vi "Config-Tab Switch.vi"(8 "error in (no error)":errorcluster, 11 "Data Cluster In":T2={"UI Reference"={"All Ctrl's Label's"=[], "ChannelListTree"=refnum, "All Object Ref"=[]}, "Tree Selection"={"Selected Channel"="", "Selected Interface"="", "Selected HW"="", "Tree Root Name"="", "Selected Module"=""}, "Selected File Path"=path "", "Selected HW"={"Slctd Hw Name"=[], "Slctd HW IP"=[]}, "Channel Config Path"=path "", "Interface Data"={"DO Channel's"=[]}, "General Info's"={"Idnentification name"=""}, "Status"="", "Channel Type's"={"Channel Type"=enum."Voltage", "Sub-Type"=enum."Pressure"}, "This VI"=refnum, "Hardware Information "=variant(variant[] [])}) -> (0 "error out":errorcluster, 2 "Config":T1(ring), 3 "Data Cluster Out":T2={"UI Reference"={"All Ctrl's Label's"=[], "ChannelListTree"=refnum, "All Object Ref"=[]}, "Tree Selection"={"Selected Channel"="", "Selected Interface"="", "Selected HW"="", "Tree Root Name"="", "Selected Module"=""}, "Selected File Path"=path "", "Selected HW"={"Slctd Hw Name"=[], "Slctd HW IP"=[]}, "Channel Config Path"=path "", "Interface Data"={"DO Channel's"=[]}, "General Info's"={"Idnentification name"=""}, "Status"="", "Channel Type's"={"Channel Type"=enum."Voltage", "Sub-Type"=enum."Pressure"}, "This VI"=refnum, "Hardware Information "=variant(variant[] [])})   [LabVIEW 2021, in "Configuration.lvlib"]
doc: "<b>Note:</b> This VI was modified by the <b>Validate DQMH Module</b> tool to turn off automatic error handling."
uses:
  Configuration.lvlib
  Module Data--cluster.ctl
  Host-Control's/Configuration UI Reference.ctl
  DO Channel's.ctl
  Config-Channel Type.ctl
  Channel Sub-Type.ctl
  <vilib>/Utility/error.llb/Clear Errors.vi
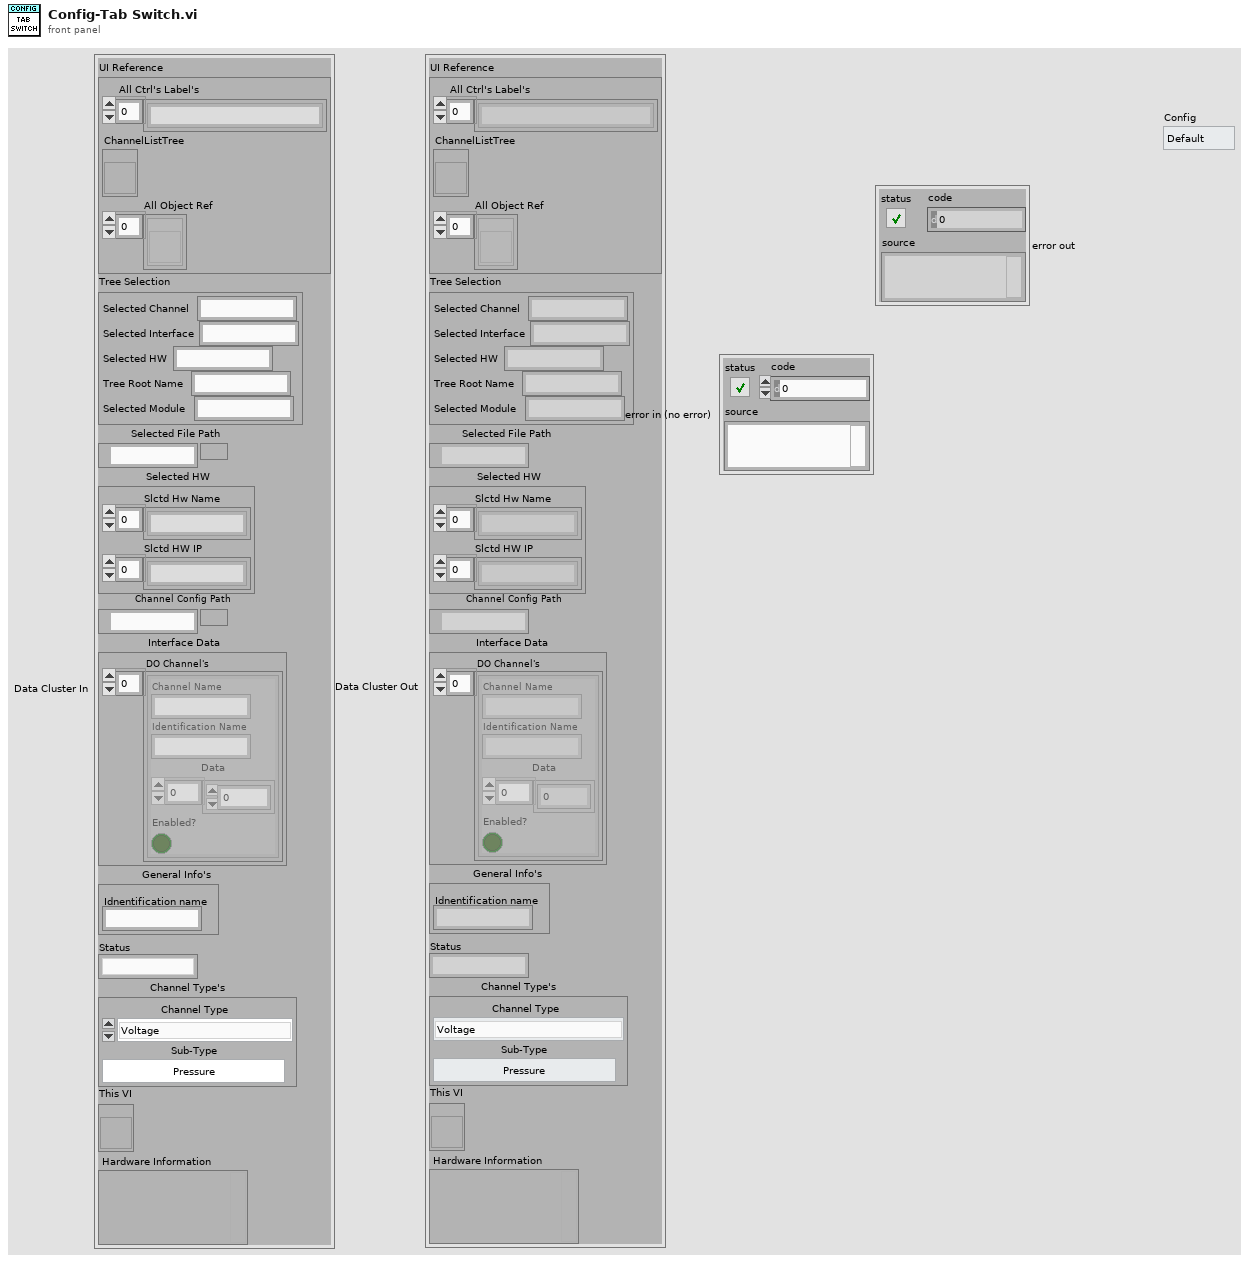
[diagram p1: front panel]
types:
  T1 = enum32{"Default", "Analog Input", "Analog Output", "Digital Input", "Digital Output", "Counter Input", "Counter Output"}
  T2 = typedef "Configuration.lvlib/Module Data--cluster.ctl" = cluster{"UI Reference":T3, "Tree Selection":cluster{"Selected Channel":string, "Selected Interface":string, "Selected HW":string, "Tree Root Name":string, "Selected Module":string}, "Selected File Path":path, "Selected HW":cluster{"Slctd Hw Name":string[], "Slctd HW IP":string[]}, "Channel Config Path":path, "Interface Data":cluster{"DO Channel's":T4}, "General Info's":cluster{"Idnentification name":string}, "Status":string, "Channel Type's":cluster{"Channel Type":T5, "Sub-Type":T6}, "This VI":refnum<vi>, "Hardware Information ":variant}
  T3 = typedef "Configuration UI Reference.ctl" = cluster{"All Ctrl's Label's":string[], "ChannelListTree":refnum<vi>, "All Object Ref":refnum<vi>[]}
  T4 = typedef "Configuration.lvlib/DO Channel's.ctl" = cluster{"Channel Name":string, "Identification Name":string, "Data":u8[], "Enabled?":bool}[]
  T5 = typedef "Configuration.lvlib/Config-Channel Type.ctl" = enum16{"Voltage", "Current", "Thermocouple", "Acclerometer"}
  T6 = typedef "Configuration.lvlib/Channel Sub-Type.ctl" = enum16{"None", "Pressure", "Force"}
  T7 = enum32{"Default", "AI-Voltage", "AI-Current", "AI-ThermoCouple", "AI-Acclerometer"}
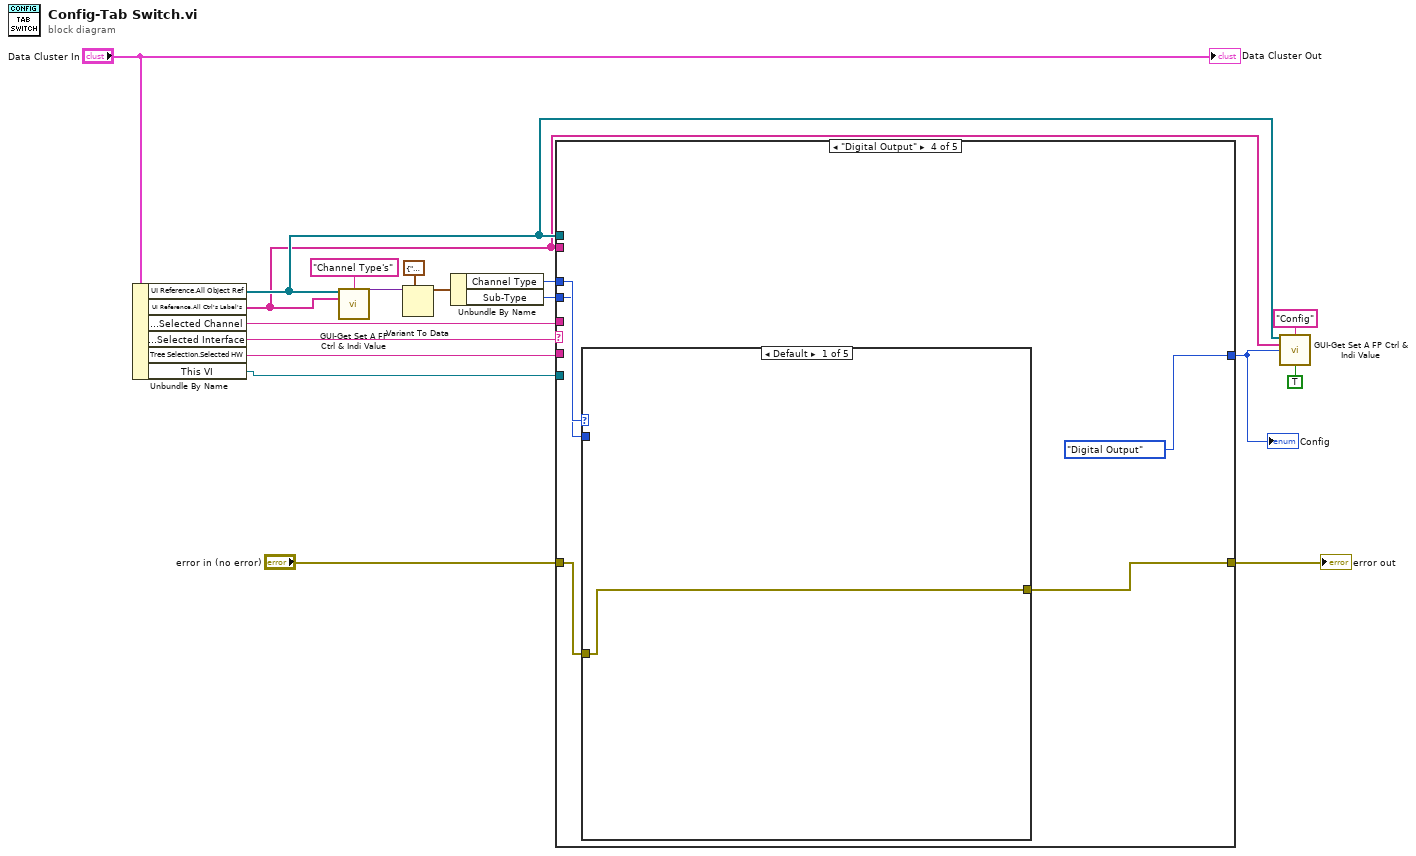
[diagram p0: block diagram]
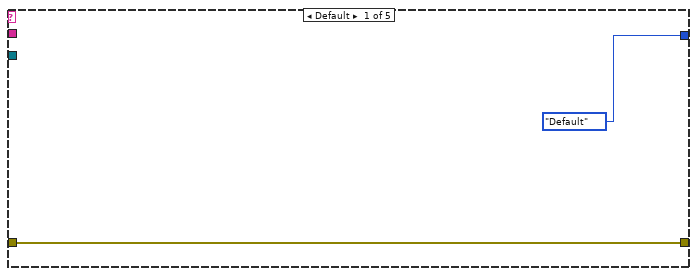
[diagram p2: hidden frame]
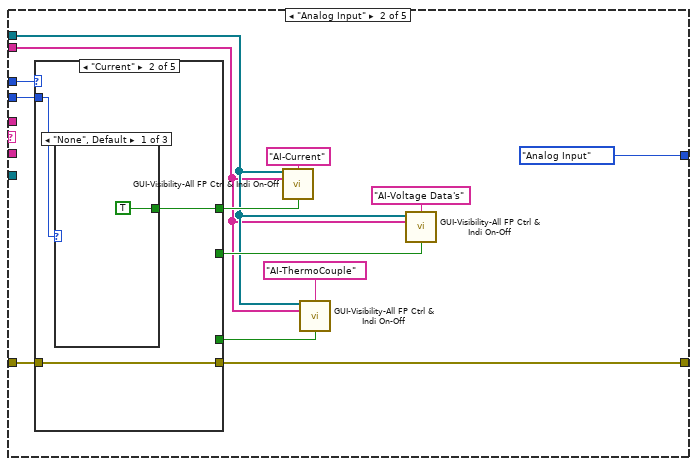
[diagram p3: hidden frame]
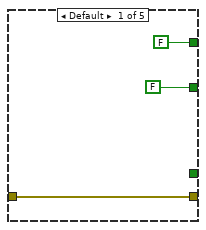
[diagram p4: hidden frame]
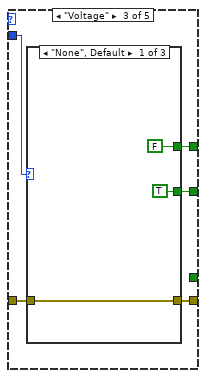
[diagram p7: hidden frame]
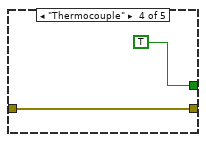
[diagram p10: hidden frame]
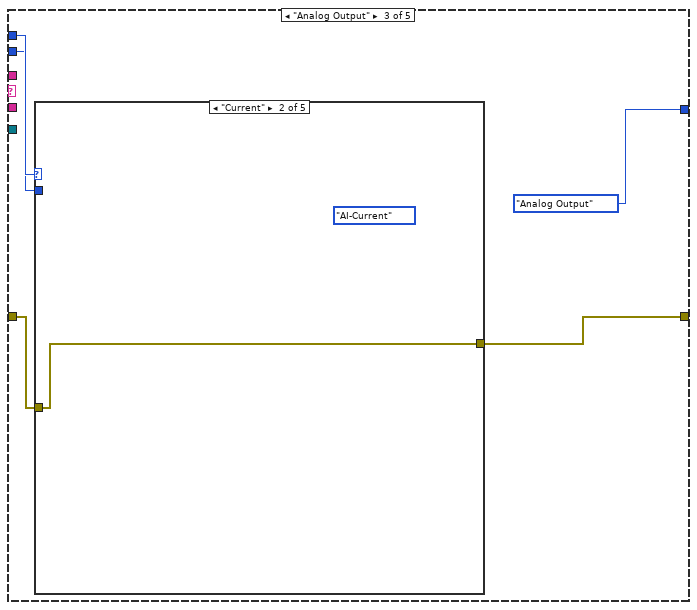
[diagram p12: hidden frame]
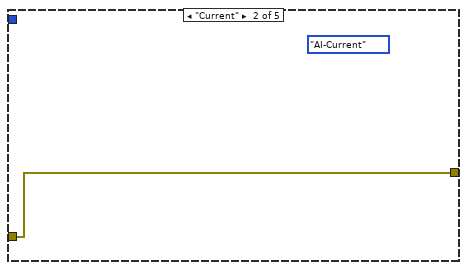
[diagram p19: hidden frame]
diagram:
  n1 = Unbundle By Name("Data Cluster In") -> ("UI Reference.All Object Ref"=w2:refnum<vi>[], "UI Reference.All Ctrl's Label's"=w1:string[], "Tree Selection.Selected Channel"=w15:string, "Tree Selection.Selected Interface"=w17:string, "Tree Selection.Selected HW"=w16:string, "This VI"=w8:refnum<vi>)
  n2 = call "GUI-Get Set A FP Ctrl & Indi Value.vi"("All Object Ref"=w2, "Label"="Channel Type's" ("Label In"), "All Object Label"=w1) -> ("Ctrl Value Out"=w3:variant)  [unwired: 9 in, 3 out]
  n3 = Variant To Data(type=cluster{"Channel Type":T5, "Sub-Type":T6} {"Channel Type"=enum."Voltage", "Sub-Type"=enum."None"} ("NewVal"), Variant=w3) -> (data=w11:cluster{"Channel Type":T5, "Sub-Type":T6})  [unwired: 1 in, 1 out]
  n4 = Unbundle By Name(w11) -> ("Channel Type"=w10:T5, "Sub-Type"=w9:T6)
  n5 = case shown="\"Digital Output\"" w17 {
    tunnel: w10 -> [_ w33 w58 w73 w88]
    tunnel: w9 -> [_ w32 w57 w72 w87]
    tunnel: w16 -> [_ _ _ _ _]
    tunnel: w15 -> [_ _ _ _ _]
    tunnel: [w20 w31 w56 w71 w86] -> w14
    tunnel: "error in (no error)" -> [w20 w30 w55 w70 w85]
    tunnel: [T1."Default" ("Config") T1."Analog Input" ("Config") T1."Analog Output" ("Config") T1."Digital Output" ("Config") T1."Digital Input" ("Config")] -> w5
    tunnel: w8 -> [_ _ _ _ _]
    tunnel: w2 -> [_ w22 _ _ _]
    tunnel: w1 -> [_ w21 _ _ _]
    frame Default {
    }
    frame "Analog Input" {
      n6 = case shown="\"Current\"" w33 {
        tunnel: w32 -> [_ w37 w45 _ _]
        tunnel: [w36 w39 w44 w52 w53] -> w31
        tunnel: w30 -> [w36 w39 w43 w52 w53]
        tunnel: [FALSE ("Visible") w38 w41 _ _] -> w27
        tunnel: [FALSE ("Visible") _ w42 _ _] -> w25
        tunnel: [_ _ _ TRUE ("Visible") _] -> w23
        frame Default {
        }
        frame "Current" {
          n7 = case shown="\"None\", Default" w37 {
            tunnel: [TRUE ("Visible") _ _] -> w38
            frame "None", Default {
            }
            frame "Pressure" {
            }
            frame "Force" {
            }
          }
        }
        frame "Voltage" {
          n8 = case shown="\"None\", Default" w45 {
            tunnel: [w48 w49 w50] -> w44
            tunnel: w43 -> [w48 w49 w50]
            tunnel: [TRUE ("Visible") _ _] -> w42
            tunnel: [FALSE ("Visible") _ _] -> w41
            frame "None", Default {
            }
            frame "Pressure" {
            }
            frame "Force" {
            }
          }
        }
        frame "Thermocouple" {
        }
        frame "Acclerometer" {
        }
      }
      n9 = call "GUI-Visibility-All FP Ctrl & Indi On-Off.vi"("All Object Ref"=w22, "Label In"="AI-Current", "All Object Label"=w21, "Visible"=w27) -> ()  [unwired: 9 in, 3 out]
      n10 = call "GUI-Visibility-All FP Ctrl & Indi On-Off.vi"("All Object Ref"=w22, "Label In"="AI-ThermoCouple", "All Object Label"=w21, "Visible"=w23) -> ()  [unwired: 9 in, 3 out]
      n11 = call "GUI-Visibility-All FP Ctrl & Indi On-Off.vi"("All Object Ref"=w22, "Label In"="AI-Voltage Data's", "All Object Label"=w21, "Visible"=w25) -> ()  [unwired: 9 in, 3 out]
    }
    frame "Analog Output" {
      n12 = case shown="\"Current\"" w58 {
        tunnel: w57 -> [_ _ w63 _ _]
        tunnel: [w59 w60 w62 w67 w68] -> w56
        tunnel: w55 -> [w59 w60 w61 w67 w68]
        frame Default {
        }
        frame "Current" {
          (unwired) T7."AI-Current" ("Value")
        }
        frame "Voltage" {
          n13 = case shown="\"None\", Default" w63 {
            tunnel: [w64 w65 w66] -> w62
            tunnel: w61 -> [w64 w65 w66]
            frame "None", Default {
            }
            frame "Pressure" {
            }
            frame "Force" {
            }
          }
        }
        frame "Thermocouple" {
        }
        frame "Acclerometer" {
        }
      }
    }
    frame "Digital Output" {
      n14 = case shown="Default" w73 {
        tunnel: w72 -> [_ _ w78 _ _]
        tunnel: [w74 w75 w77 w82 w83] -> w71
        tunnel: w70 -> [w74 w75 w76 w82 w83]
        frame Default {
        }
        frame "Current" {
          (unwired) T7."AI-Current" ("Value")
        }
        frame "Voltage" {
          n15 = case shown="\"None\", Default" w78 {
            tunnel: [w79 w80 w81] -> w77
            tunnel: w76 -> [w79 w80 w81]
            frame "None", Default {
            }
            frame "Pressure" {
            }
            frame "Force" {
            }
          }
        }
        frame "Thermocouple" {
        }
        frame "Acclerometer" {
        }
      }
    }
    frame "Digital Input" {
      n16 = case shown="Default" w88 {
        tunnel: w87 -> [_ _ w93 _ _]
        tunnel: [w89 w90 w92 w97 w98] -> w86
        tunnel: w85 -> [w89 w90 w91 w97 w98]
        frame Default {
        }
        frame "Current" {
          (unwired) T7."AI-Current" ("Value")
        }
        frame "Voltage" {
          n17 = case shown="\"None\", Default" w93 {
            tunnel: [w94 w95 w96] -> w92
            tunnel: w91 -> [w94 w95 w96]
            frame "None", Default {
            }
            frame "Pressure" {
            }
            frame "Force" {
            }
          }
        }
        frame "Thermocouple" {
        }
        frame "Acclerometer" {
        }
      }
    }
  }
  "error out" <- w14
  "Config" <- w5
  n18 = call "GUI-Get Set A FP Ctrl & Indi Value.vi"("All Object Ref"=w2, "Label"="Config" ("Label In"), "All Object Label"=w1, "Ctrl Value In"=w5, "Set(F)"=TRUE) -> ()  [unwired: 7 in, 4 out]
  "Data Cluster Out" <- "Data Cluster In"
